vi "Mini car game1.vi"() -> ()   [LabVIEW 2019]
uses:
  Supported.llb/Global-1.vi
  <vilib>/Analysis/NI_AALBase.lvlib
  <vilib>/Utility/miscctls.llb/LVPointTypeDef.ctl
panel:
  out "XY Graph":cluster{dbl[], dbl[]}[](graph)
  in  "UP":bool
  out "SCORE":dbl
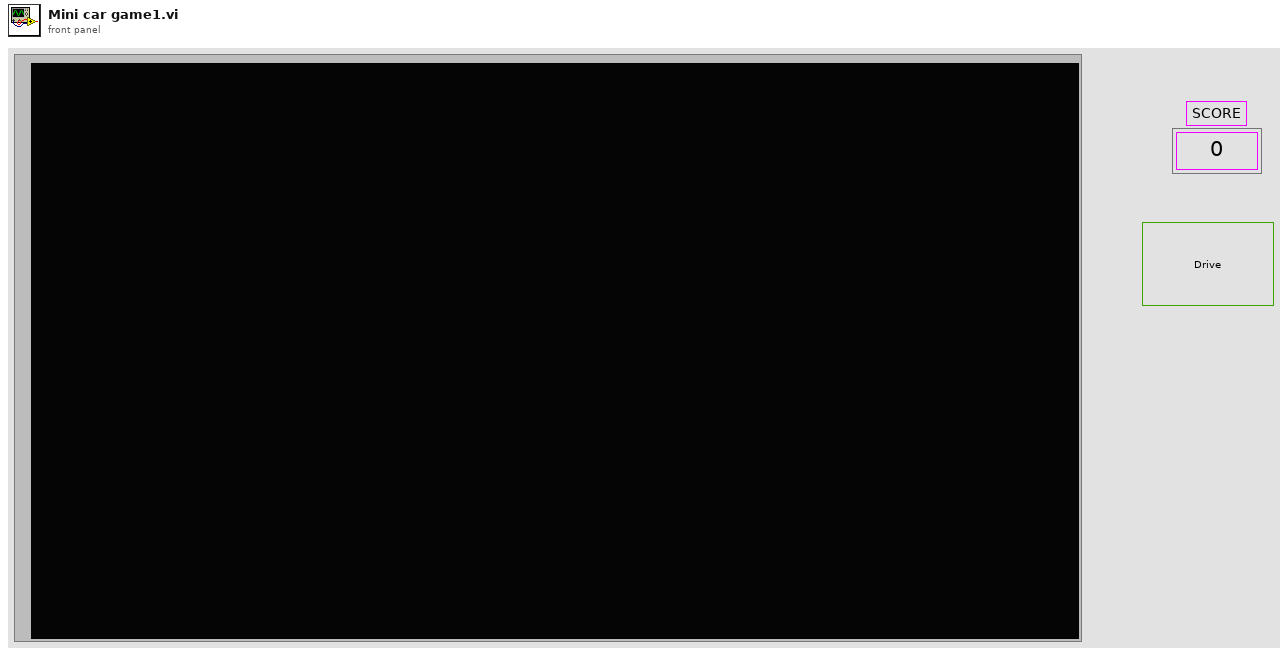
[diagram p1: front panel]
types:
  T1 = typedef "LVPointTypeDef.ctl" = cluster{"Horizontal":i16, "Vertical":i16}
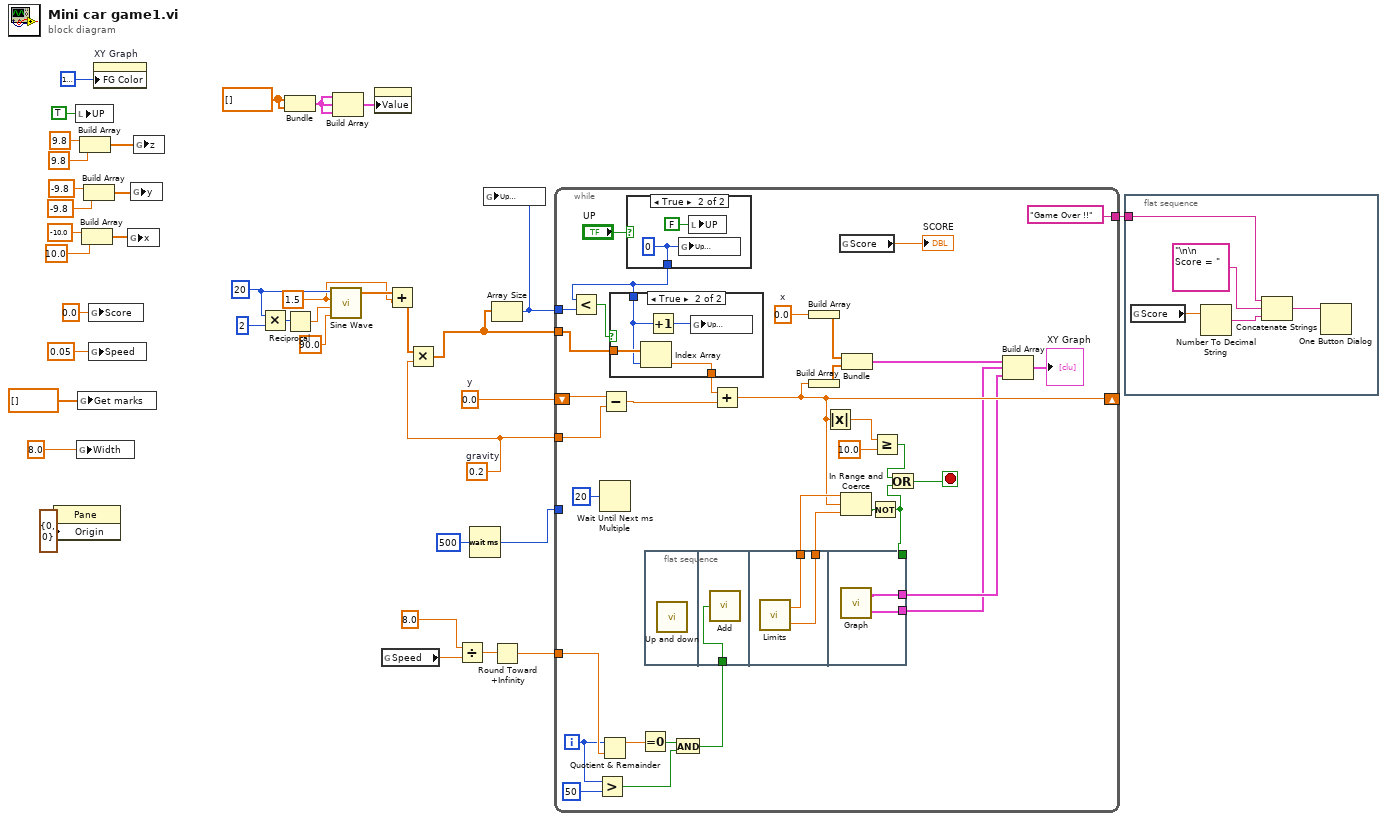
[diagram p0: block diagram]
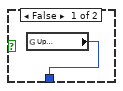
[diagram p2: hidden frame]
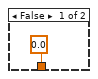
[diagram p3: hidden frame]
diagram:
  w12 = dbl[] []
  w27 = 1.5 ("amplitude")
  w36 = 20 ("samples")
  w30 = 0.2  # gravity
  w38 = 0.0  # y
  n1 = property on="Property Node" class="Pane"("Origin"=T1 {"Horizontal"=0, "Vertical"=0}) -> ()  [unwired: 2 in, 2 out]
  n2 = local write "UP"(TRUE ("UP")) -> ()
  n3 = global write "Global-1.vi" "Width"(8.0 ("opening width")) -> ()
  n4 = global write "Global-1.vi" "Get marks"(dbl[] []) -> ()
  n5 = Build Array(9.8 ("element"), 9.8 ("element")) -> (w14:dbl[])
  n6 = Build Array(-10.0 ("element"), 10.0 ("element")) -> (w16:dbl[])
  n7 = Build Array(-9.8 ("element"), -9.8 ("element")) -> (w15:dbl[])
  n8 = global write "Global-1.vi" "Score"(0.0 ("Score")) -> ()
  n9 = global write "Global-1.vi" "Speed"(0.05 ("Score")) -> ()
  n10 = property on="XY Graph" class="XYGraph (strict)"("FG Color"=u32 16777216) -> ()  [unwired: 2 in, 2 out]
  n11 = global write "Global-1.vi" "x"(w16) -> ()
  n12 = global write "Global-1.vi" "y"(w15) -> ()
  n13 = global write "Global-1.vi" "z"(w14) -> ()
  n14 = Multiply(x=w36, y=2) -> (x*y=w34:i32)
  n15 = Bundle(w12, w12) -> (w13:cluster{dbl[], dbl[]})  [unwired: 1 in]
  n16 = Reciprocal(x=w34) -> (1/x=w33:dbl)
  n17 = call <vilib>:"Sine Wave.vi"("samples"=w36, "amplitude"=w27, "frequency"=w33, "phase in"=90.0) -> ("sine wave"=w32:dbl[])  [unwired: 1 in, 2 out]
  n18 = Build Array(w13, w13, w13) -> (w26:cluster{dbl[], dbl[]}[])
  n19 = property on="XY Graph" class="XYGraph (strict)"("Value"=w26) -> ()  [unwired: 2 in, 2 out]
  n20 = global read "Global-1.vi" "Speed"() -> (w9:dbl)
  n21 = Add(x=w32, y=w27) -> (x+y=w31:dbl[])
  n22 = Multiply(x=w31, y=w30) -> (x*y=w29:dbl[])
  n23 = Divide(x=8.0, y=w9) -> (x/y=w7:dbl)
  n24 = Wait (ms)(milliseconds to wait=u32 500) -> (millisecond timer value=w24:u32)
  n25 = Array Size(array=w29) -> (size(s)=w17:i32)
  n26 = global write "Global-1.vi" "Up \nUp"(w17) -> ()
  n27 = Round Toward +Infinity(x=w7) -> (ceil(x): smallest int >= x=w6:dbl)
  n28 = while {
    tunnel: w30 -> [w66]
    shift-right: [w53] -> _
    shift-left: w38 -> [w67]
    tunnel: w29 -> [w63]
    tunnel: w17 -> [w65]
    tunnel: ["Game Over !!" ("message")] -> w5
    tunnel: w24 -> [_]
    tunnel: w6 -> [w47]
    i -> [w43]
    stop <- w39 stop-if-true
    w68 = 0.0  # x
    n29 = Greater?(x=w43, y=50) -> (0:w41:bool)
    n30 = Wait Until Next ms Multiple(millisecond multiple=u32 20) -> ()  [unwired: 1 out]
    n31 = Quotient & Remainder(x=w43, y=w47) -> (x-y*floor(x/y)=w46:dbl)  [unwired: 1 out]
    n32 = Subtract(x=w67, y=w66) -> (x-y=w62:dbl)
    n33 = case shown="True" "UP" {
      tunnel: [w79 w80] -> w59
      frame False {
        n34 = global read "Global-1.vi" "Up \nUp"() -> (w79:i32)
      }
      frame True {
        w80 = 0 ("Up index")
        n35 = global write "Global-1.vi" "Up \nUp"(w80) -> ()
        n36 = local write "UP"(FALSE ("UP")) -> ()
      }
    }
    n37 = Less?(x=w59, y=w65) -> (x < y?=w64:bool)
    n38 = case shown="True" w64 {
      tunnel: w63 -> [_ w86]
      tunnel: w59 -> [_ w85]
      tunnel: [0.0 w84] -> w61
      frame False {
      }
      frame True {
        n39 = Index Array(array=w86, index=w85) -> (element=w84:dbl)
        n40 = Increment(x=w85) -> (x+1=w83:i32)
        n41 = global write "Global-1.vi" "Up \nUp"(w83) -> ()
      }
    }
    n42 = Equal To 0?(x=w46) -> (x = 0?=w45:bool)
    n43 = flat-sequence {
      tunnel: w44 -> [w74]
      tunnel: [w76] -> w55
      tunnel: [w75] -> w54
      tunnel: [w77] -> w50
      tunnel: [w78] -> w49
      tunnel: w48 -> [_]
      frame #0 {
        n44 = call "Up and down.vi"() -> ()  [unwired: 12 in]
      }
      frame #1 {
        n45 = call "Add.vi"("Add"=w74) -> ()
      }
      frame #2 {
        n46 = call "Limits.vi"() -> ("lower limit"=w75:dbl, "upper limit"=w76:dbl)  [unwired: 2 in]
      }
      frame #3 {
        n47 = call "Graph.vi"() -> ("Lower"=w78:cluster{"x":dbl[], "y":dbl[]}, "Upper"=w77:cluster{"x":dbl[], "z":dbl[]})  [unwired: 2 in]
      }
    }
    n48 = And(x=w45, y=w41) -> (x .and. y?=w44:bool)
    n49 = Add(x=w61, y=w62) -> (x+y=w53:dbl)
    n50 = Build Array(w68) -> (w70:dbl[])
    n51 = Build Array(w53) -> (w69:dbl[])
    n52 = Absolute Value(x=w53) -> (abs(x)=w71:dbl)
    n53 = global read "Global-1.vi" "Score"() -> (→"SCORE":dbl)
    n54 = In Range and Coerce(upper limit=w55, x=w53, lower limit=w54) -> (In Range?=w51:bool)  [unwired: 1 out]
    n55 = Bundle(w70, w69) -> (w58:cluster{dbl[], dbl[]})  [unwired: 1 in]
    n56 = Not(x=w51) -> (.not. x?=w48:bool)
    n57 = Greater Or Equal?(x=w71, y=10.0) -> (x >= y?=w52:bool)
    n58 = Or(x=w52, y=w48) -> (x .or. y?=w39:bool)
    n59 = Build Array(w58, w49, w50) -> (→"XY Graph":cluster{"x":dbl[], "z":dbl[]}[])
  }
  n60 = flat-sequence {
    tunnel: w5 -> [w87]
    frame #0 {
      n61 = global read "Global-1.vi" "Score"() -> (w91:dbl)
      n62 = Number To Decimal String(number=w91) -> (decimal integer string=w90:string)  [unwired: 1 in]
      n63 = Concatenate Strings(w87, "\n\n  Score = " ("string"), w90) -> (w88:string)
      n64 = One Button Dialog(message=w88) -> ()  [unwired: 1 in, 1 out]
    }
  }
